vi "WriteToDb.vi"(0 "reference in":refnum<class "AI.lvclass">, 11 "error in (no error)":errorcluster) -> (4 "reference out":refnum<class "AI.lvclass">, 15 "error out":errorcluster)   [LabVIEW 2019, in "AI.lvclass"]
uses:
  AI.lvclass
  C:/Users/ANENKOV_V1/Desktop/src/Proccess_class/Proccess.lvclass
  AI.lvclass/AI.ctl
  Proccess_class/Proccess.lvclass/Proccess.ctl
  Logger_class/SignalData.ctl
  Logger_class/Logger.lvclass/Logger.ctl
  Logger_class/Logger.lvclass
  Proccess_class/Proccess.lvclass
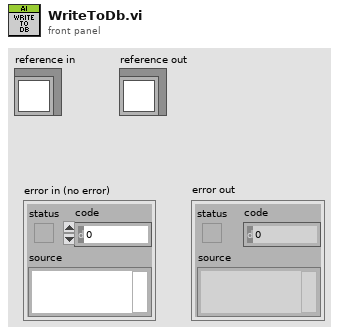
[diagram p1: front panel]
types:
  T1 = typedef "Logger.lvclass/SignalData.ctl" = cluster{"Value":dbl, "SignalTag":string, "ObjTag":string, "Desc":string, "Time Stamp":timestamp}
  T2 = typedef "Proccess.lvclass/TAGs.ctl" = cluster{"TAG":string, "PTAG":string, "DESC":string}
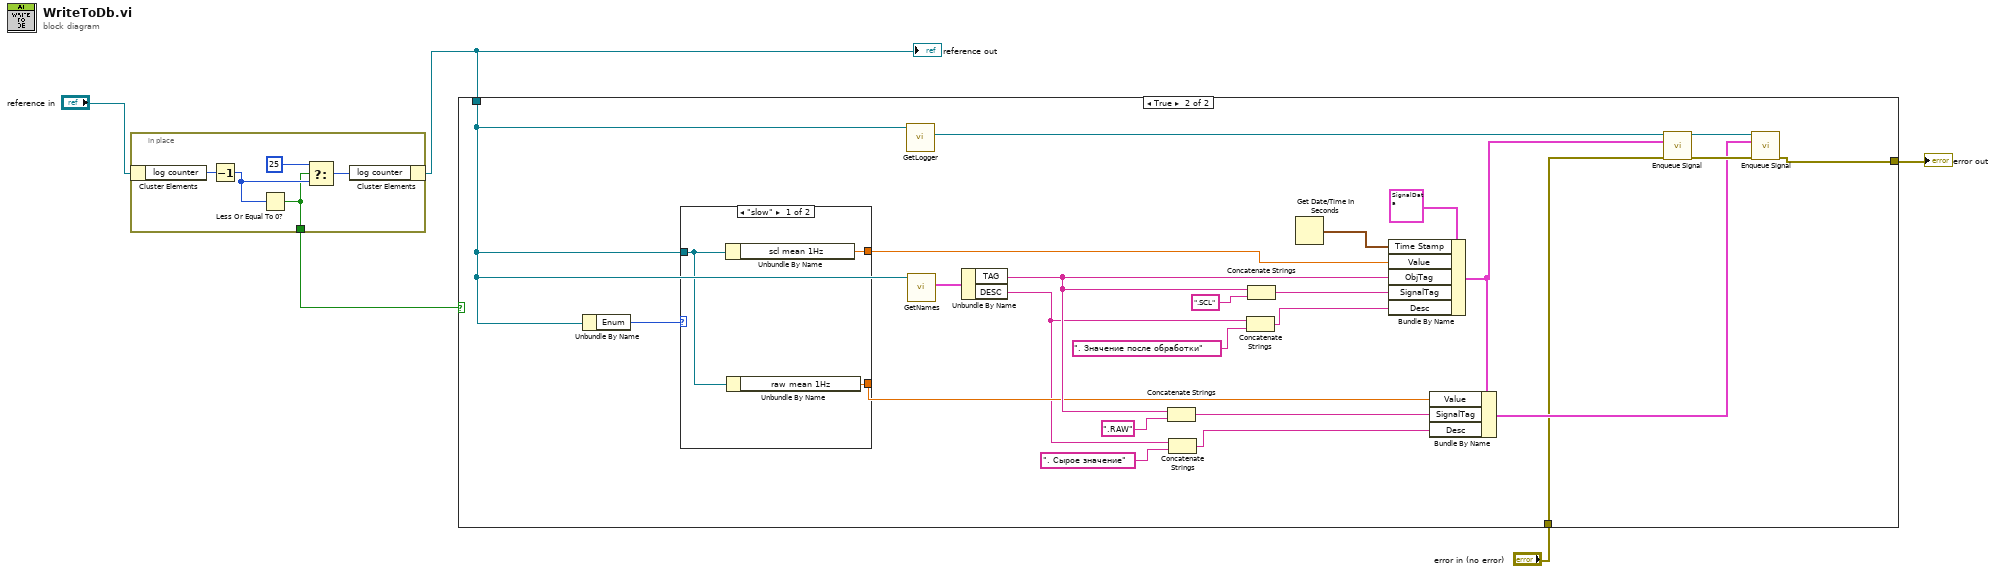
[diagram p0: block diagram]
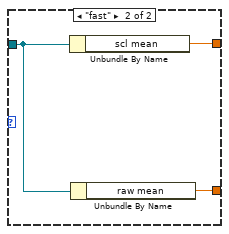
[diagram p3: hidden frame]
diagram:
  n1 = in-place {
    in-place-border: [w6] -> w1
    n2 = in-place-cluster #1("reference in") -> ("log counter"=w10:i32)
    n3 = Decrement(x=w10) -> (x-1=w7:i32)
    n4 = Less Or Equal To 0?(x=w7) -> (x <= 0?=w6:bool)
    n5 = Select(t=25, s=w6, f=w7) -> (s? t:f=w8:i32)
    n6 = in-place-cluster #1("log counter"=w8) -> (w4:refnum<class "AI.lvclass">)
  }
  "reference out" <- w4
  n7 = case shown="True" w1 {
    tunnel: w4 -> [_ w14]
    tunnel: "error in (no error)" -> [w11 w13]
    tunnel: [w11 w12] -> w2
    frame False {
    }
    frame True {
      n8 = Unbundle By Name(w14) -> ("Enum"=w15:enum16{"fast", "slow"})
      n9 = case shown="\"slow\"" w15 {
        tunnel: [w38 w41] -> w32
        tunnel: [w37 w40] -> w20
        tunnel: w14 -> [w36 w39]
        frame "slow" {
          n10 = Unbundle By Name(w36) -> ("scl mean 1Hz"=w38:dbl)
          n11 = Unbundle By Name(w36) -> ("raw mean 1Hz"=w37:dbl)
        }
        frame "fast" {
          n12 = Unbundle By Name(w39) -> ("scl mean"=w41:dbl)
          n13 = Unbundle By Name(w39) -> ("raw mean"=w40:dbl)
        }
      }
      n14 = call "GetLogger.vi"("Proccess in"=w14) -> ("Logger"=w25:refnum<class "Logger.lvclass">)  [unwired: 10 in]
      n15 = call "GetNames.vi"("Proccess in"=w14) -> ("Tags"=w26:T2)  [unwired: 10 in]
      n16 = Unbundle By Name(w26) -> ("TAG"=w24:string, "DESC"=w17:string)
      n17 = Concatenate Strings(w24, ".RAW" ("string")) -> (w18:string)
      n18 = Concatenate Strings(w17, ". Сырое значение" ("string")) -> (w16:string)
      n19 = Concatenate Strings(w17, ". Значение после обработки" ("string")) -> (w21:string)
      n20 = Concatenate Strings(w24, ".SCL" ("string")) -> (w33:string)
      n21 = Get Date/Time In Seconds() -> (seconds since 1Jan1904=w23:timestamp)
      n22 = Bundle By Name(cluster=T1 {"Value"=0.0, "SignalTag"="", "ObjTag"="", "Desc"="", "Time Stamp"=timestamp(0 s since 1904-01-01)} ("element"), "Time Stamp"=w23, "Value"=w32, "ObjTag"=w24, "SignalTag"=w33, "Desc"=w21) -> (w29:T1)
      n23 = Bundle By Name(cluster=w29, "Value"=w20, "SignalTag"=w18, "Desc"=w16) -> (w27:T1)
      n24 = call "Enqueue Signal.vi"("reference in"=w25, "element"=w29, "error in (no error)"=w13) -> ("reference out"=w31:refnum<class "Logger.lvclass">, "error out"=w30:errorcluster)  [unwired: 11 in]
      n25 = call "Enqueue Signal.vi"("reference in"=w31, "element"=w27, "error in (no error)"=w30) -> ("error out"=w12:errorcluster)  [unwired: 11 in, 1 out]
    }
  }
  "error out" <- w2
